vi "Synth Get Amplitude Clock.vi"(1 "Clk String Lngth":i8=40) -> (0 "TimingClock":u8[](array[numeric]) format="%08b")   [LabVIEW 2015]
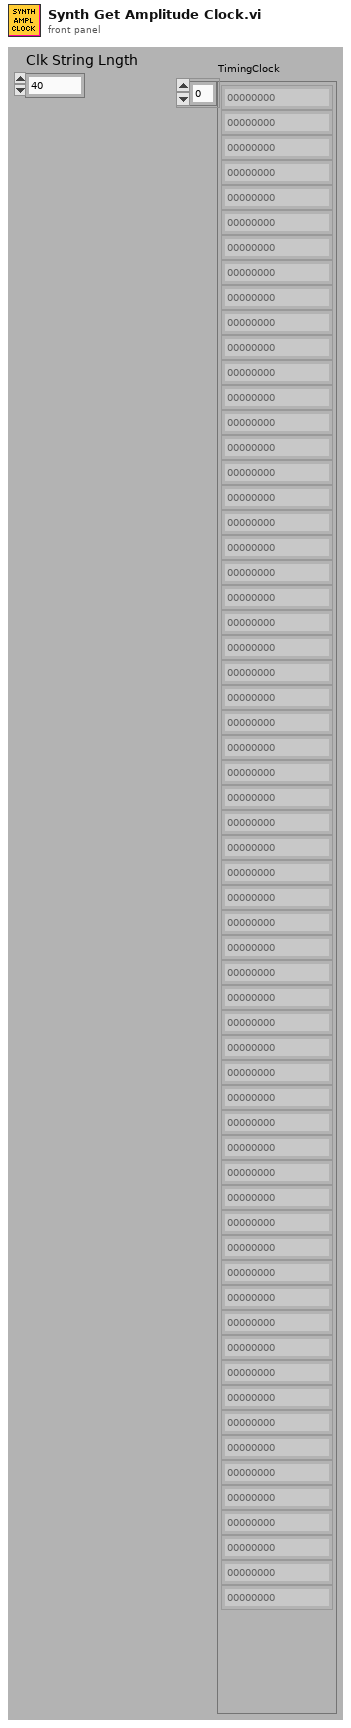
[diagram p1: front panel]
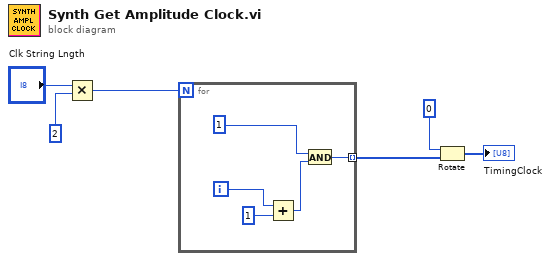
[diagram p0: block diagram]
diagram:
  n1 = Multiply(x="Clk String Lngth", y=2) -> (x*y=w5:i32)
  n2 = for {
    N: w5 -> [_]
    tunnel: [w11] -> w2 mode=indexing
    i -> [w8]
    n3 = Add(x=w8, y=u8 1) -> (x+y=w7:i32)
    n4 = And(x=1, y=w7) -> (x .and. y?=w11:i32)
  }
  n5 = Rotate(1:w2, 2:0) -> (0:→"TimingClock":i32[])
